vi "LV SciSDK LIST START.vi"(0 "List name":string, 1 "Acq Len":u32=1024, 2 "Acq Mode":string(combo)="blocking", 3 "Timeout":i32=100, 4 "Handle In":T1, 5 "error in (no error)":errorcluster, 6 "Thread":string(combo)="false", 8 "High Performance":string(combo)="false", 10 "Threaded Buffer Size":u32=100000) -> (17 "CP Handle Out":cluster{"CP Path":string, "CP Name":string}, 18 "Handle Out":T1, 19 "error out":errorcluster)   [LabVIEW 2021, in "SciSDK_Labview.lvlib"]
uses:
  SciSDK_Labview.lvlib
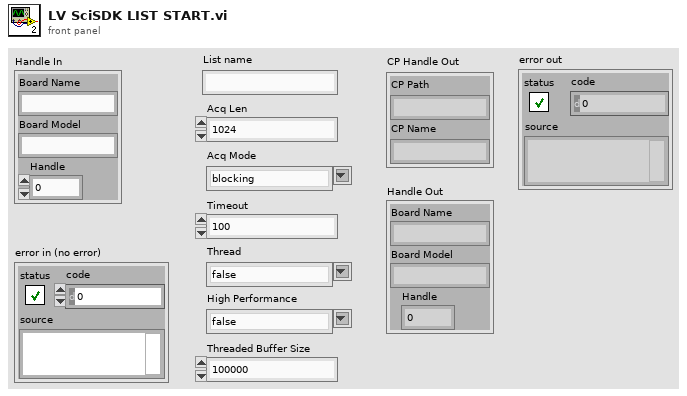
[diagram p1: front panel]
types:
  T1 = cluster{"Board Name":string, "Board Model":string, "Handle":u64}
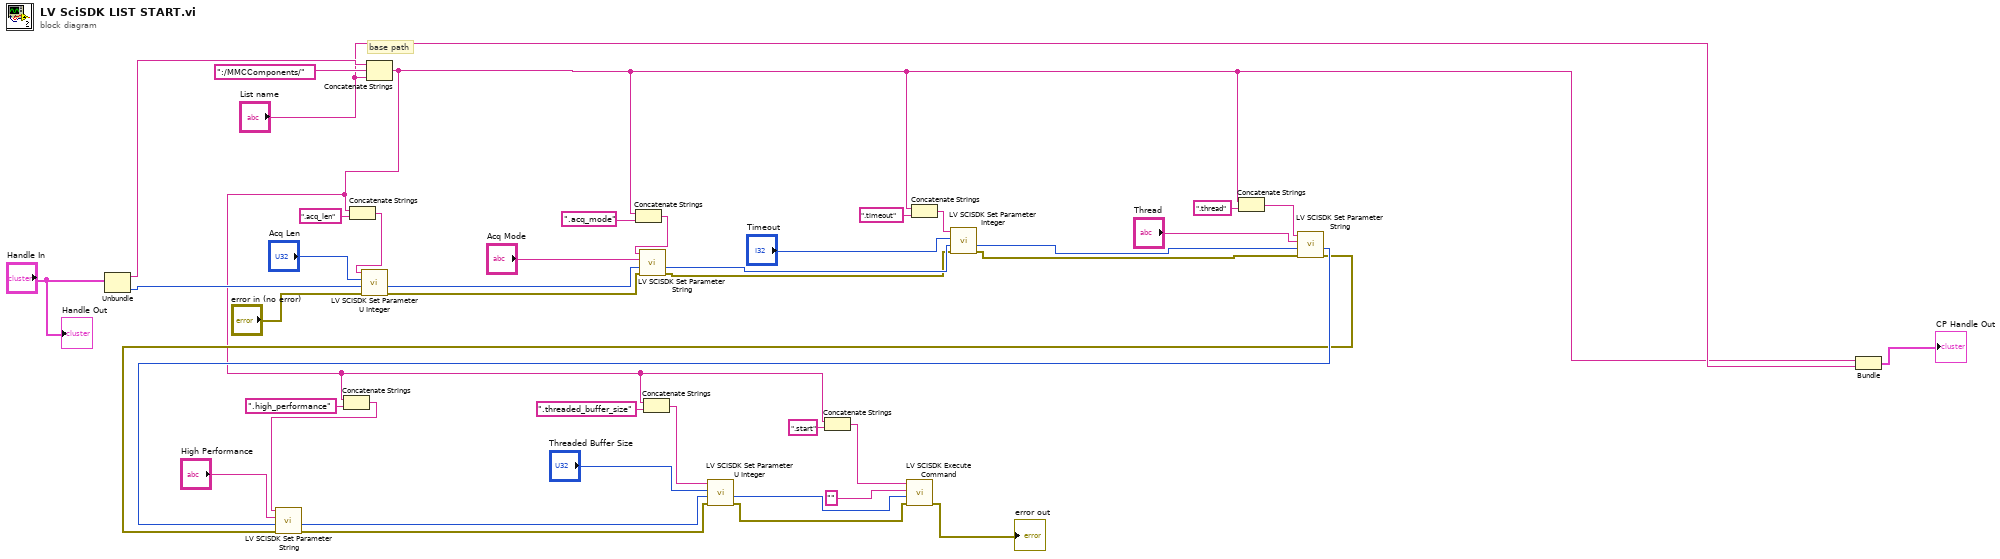
[diagram p0: block diagram]
diagram:
  # "base path"
  n1 = Unbundle("Handle In") -> ("Board Name"=w41:string, "Handle"=w28:u64)  [unwired: 1 out]
  n2 = Concatenate Strings(w41, ":/MMCComponents/" ("string"), "List name") -> (w2:string)
  n3 = Concatenate Strings(w2, ".high_performance" ("string")) -> (w15:string)
  n4 = Concatenate Strings(w2, ".acq_len" ("string")) -> (w30:string)
  n5 = call "LV SCISDK Set Parameter U Integer.vi"("error in (no error)"="error in (no error)", "handle"=w28, "value"="Acq Len", "Path"=w30) -> ("error out"=w25:errorcluster, "handle out"=w26:u64)  [unwired: 5 in, 1 out]
  n6 = Concatenate Strings(w2, ".acq_mode" ("string")) -> (w32:string)
  n7 = call "LV SCISDK Set Parameter String.vi"("error in (no error)"=w25, "handle"=w26, "value"="Acq Mode", "Path"=w32) -> ("error out"=w21:errorcluster, "handle out"=w22:u64)  [unwired: 5 in, 1 out]
  n8 = Concatenate Strings(w2, ".threaded_buffer_size" ("string")) -> (w12:string)
  n9 = Concatenate Strings(w2, ".start" ("string")) -> (w5:string)
  n10 = Concatenate Strings(w2, ".timeout" ("string")) -> (w24:string)
  n11 = call "LV SCISDK Set Parameter Integer.vi"("error in (no error)"=w21, "handle"=w22, "value"="Timeout", "Path"=w24) -> ("error out"=w17:errorcluster, "handle out"=w18:u64)  [unwired: 5 in, 1 out]
  n12 = Concatenate Strings(w2, ".thread" ("string")) -> (w19:string)
  n13 = call "LV SCISDK Set Parameter String.vi"("error in (no error)"=w17, "handle"=w18, "value"="Thread", "Path"=w19) -> ("error out"=w13:errorcluster, "handle out"=w14:u64)  [unwired: 5 in, 1 out]
  n14 = call "LV SCISDK Set Parameter String.vi"("error in (no error)"=w13, "handle"=w14, "value"="High Performance", "Path"=w15) -> ("error out"=w9:errorcluster, "handle out"=w10:u64)  [unwired: 5 in, 1 out]
  n15 = call "LV SCISDK Set Parameter U Integer.vi"("error in (no error)"=w9, "handle"=w10, "value"="Threaded Buffer Size", "Path"=w12) -> ("error out"=w8:errorcluster, "handle out"=w3:u64)  [unwired: 5 in, 1 out]
  n16 = call "LV SCISDK Execute Command.vi"("error in (no error)"=w8, "handle"=w3, "value"="", "Path"=w5) -> ("error out"=→"error out":errorcluster)  [unwired: 5 in, 2 out]
  n17 = Bundle(w2, "List name"="List name") -> (→"CP Handle Out":cluster{string, "List name":string})  [unwired: 1 in]
  "Handle Out" <- "Handle In"
